vi "main_load_environment_check.vi"(10 "New working Dir":path) -> (1 "Structure":string, 2 "Valid?":bool, 3 "Endtime":string)   [LabVIEW 2019]
uses:
  <vilib>/regexp/Match Regular Expression.xnode
panel:
  out "Starttime":string
  out "Finished?":string
  out "Timesteps":i32[](array[numeric])
  # "*******************************************************************\nBiogas Plant Control\n\nAuthor: Paul Zügel\nGCSC-Frankfurt am Main 2020\n\n*******************************************************************"
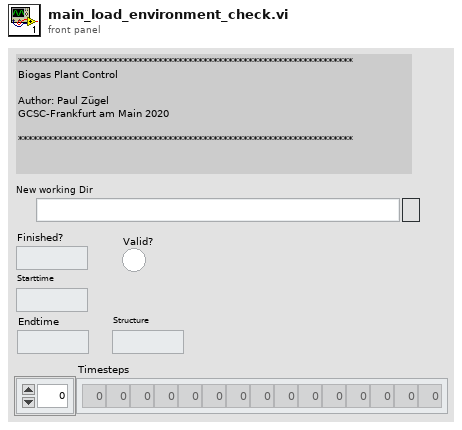
[diagram p1: front panel]
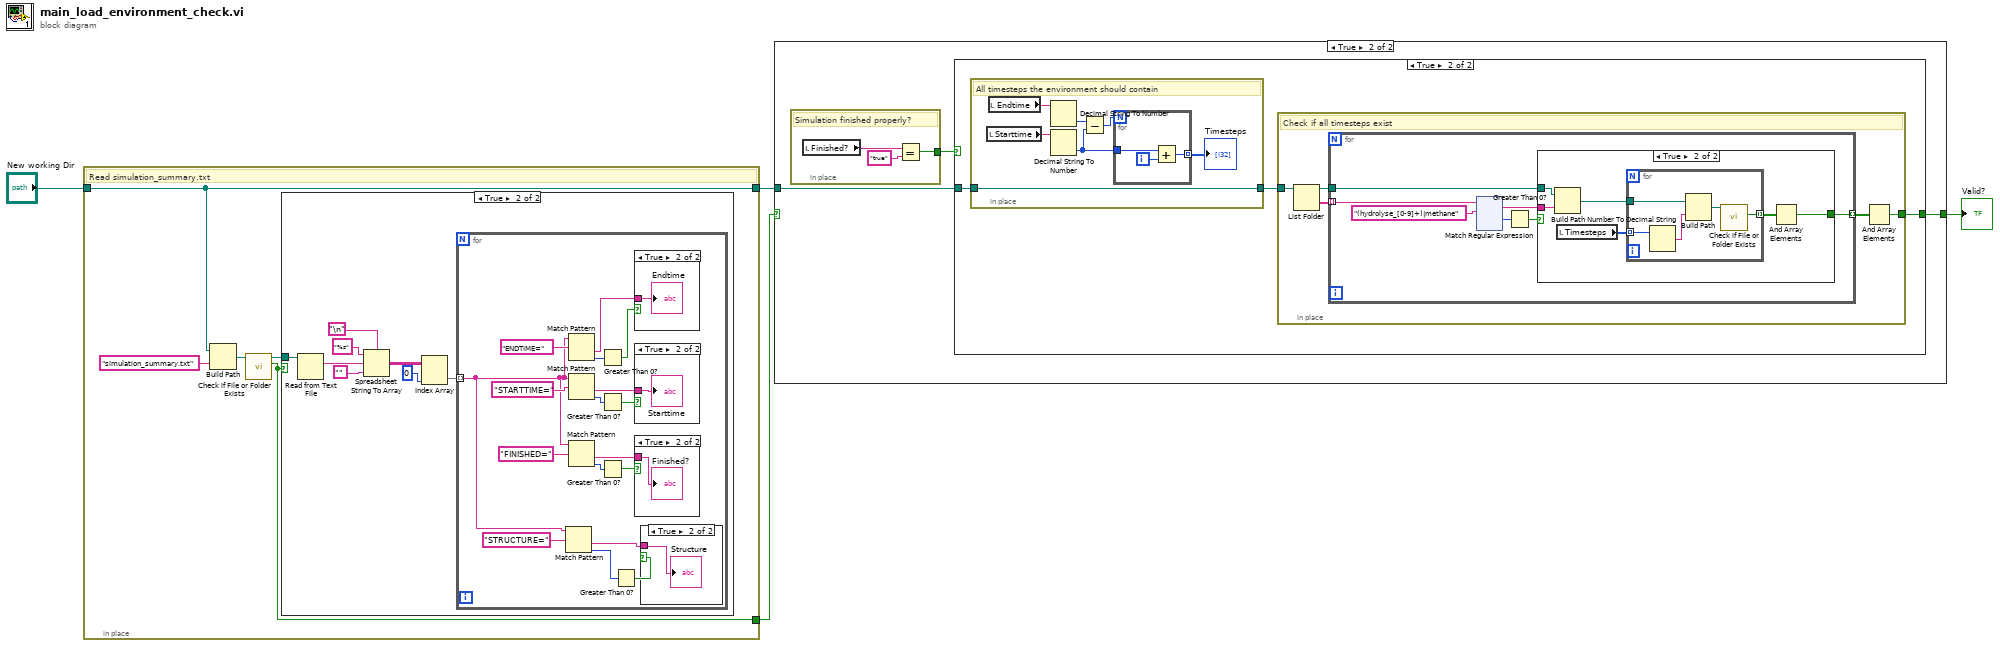
[diagram p0: block diagram]
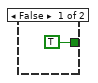
[diagram p4: hidden frame]
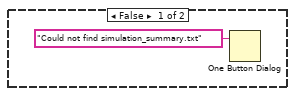
[diagram p5: hidden frame]
diagram:
  n1 = in-place {
    in-place-border: [w7] -> w1
    in-place-border: "New working Dir" -> [w5]
    in-place-border: [w5] -> w2
    # "Read simulation_summary.txt"
    n2 = Build Path(base path=w5, name or relative path="simulation_summary.txt") -> (appended path=w6:path)
    n3 = call <vilib>:"Check if File or Folder Exists.vi"("path"=w6) -> ("file or folder exists?"=w7:bool, "dup path"=w8:path)  [unwired: 8 in, 1 out]
    n4 = case shown="True" w7 {
      tunnel: w8 -> [_ w18]
      frame False {
        n5 = One Button Dialog(message="Could not find simulation_summary.txt") -> ()  [unwired: 1 in, 1 out]
      }
      frame True {
        n6 = Read from Text File(file (use dialog)=w18) -> (text=w17:string)  [unwired: 3 in, 3 out]
        n7 = Spreadsheet String To Array(delimiter (Tab)="\n", format string="%s", spreadsheet string=w17, array type (2D Dbl)="") -> (array=w11:string[][])
        n8 = Index Array(array=w11, index (col)=0 ("disabled index (col)")) -> (element=w12:string[])  [unwired: 1 in]
        n9 = for {
          tunnel: w12 -> [w19] mode=indexing
          n10 = Match Pattern(string=w19, regular expression="STRUCTURE=") -> (after substring=w22:string, offset past match=w21:i32)  [unwired: 1 in, 2 out]
          n11 = Match Pattern(string=w19, regular expression="ENDTIME=") -> (after substring=w30:string, offset past match=w25:i32)  [unwired: 1 in, 2 out]
          n12 = Match Pattern(string=w19, regular expression="STARTTIME=") -> (after substring=w32:string, offset past match=w27:i32)  [unwired: 1 in, 2 out]
          n13 = Match Pattern(string=w19, regular expression="FINISHED=") -> (after substring=w34:string, offset past match=w29:i32)  [unwired: 1 in, 2 out]
          n14 = Greater Than 0?(x=w25) -> (x > 0?=w24:bool)
          n15 = Greater Than 0?(x=w27) -> (x > 0?=w26:bool)
          n16 = Greater Than 0?(x=w29) -> (x > 0?=w28:bool)
          n17 = Greater Than 0?(x=w21) -> (x > 0?=w20:bool)
          n18 = case shown="True" w24 {
            tunnel: w30 -> [_ w39]
            frame False {
            }
            frame True {
              "Endtime" <- w39
            }
          }
          n19 = case shown="True" w26 {
            tunnel: w32 -> [_ w38]
            frame False {
            }
            frame True {
              "Starttime" <- w38
            }
          }
          n20 = case shown="True" w28 {
            tunnel: w34 -> [_ w37]
            frame False {
            }
            frame True {
              "Finished?" <- w37
            }
          }
          n21 = case shown="True" w20 {
            tunnel: w22 -> [_ w36]
            frame False {
            }
            frame True {
              "Structure" <- w36
            }
          }
        }
      }
    }
  }
  n22 = case shown="True" w1 {
    selector: w1 -> [w40 _]
    tunnel: [w40 w43] -> w4
    tunnel: w2 -> [_ w42]
    frame False {
    }
    frame True {
      n23 = in-place {
        in-place-border: [w196] -> w41
        # "Simulation finished properly?"
        n24 = local read "Finished?"() -> (w198:string)
        n25 = Equal?(x=w198, y="true") -> (x = y?=w196:bool)
      }
      n26 = case shown="True" w41 {
        selector: w41 -> [w44 _]
        tunnel: [w44 w47] -> w43
        tunnel: w42 -> [_ w45]
        frame False {
        }
        frame True {
          n27 = in-place {
            in-place-border: w45 -> [w50]
            in-place-border: [w50] -> w46
            # "All timesteps the environment should contain"
            n28 = local read "Starttime"() -> (w48:string)
            n29 = local read "Endtime"() -> (w49:string)
            n30 = Decimal String To Number(string=w49) -> (number=w54:i32)  [unwired: 2 in, 1 out]
            n31 = Decimal String To Number(string=w48) -> (number=w52:i32)  [unwired: 2 in, 1 out]
            n32 = Subtract(x=w54, y=w52) -> (x-y=w53:i32)
            n33 = for {
              N: w53 -> [_]
              tunnel: w52 -> [w56]
              tunnel: [w55] -> w51 mode=indexing
              i -> [w57]
              n34 = Add(x=w56, y=w57) -> (x+y=w55:i32)
            }
            "Timesteps" <- w51
          }
          n35 = in-place {
            in-place-border: [w62] -> w47
            in-place-border: w46 -> [w61]
            # "Check if all timesteps exist"
            n36 = List Folder(path=w61) -> (path out=w59:path, folder names=w60:string[])  [unwired: 3 in, 2 out]
            n37 = for {
              tunnel: w60 -> [w68] mode=indexing
              tunnel: w59 -> [w65]
              tunnel: [w63] -> w58 mode=indexing
              n38 = xnode "Match Regular Expression"("input string"=w68, "regular expression"="(hydrolyse_[0-9]+)|methane") -> ("whole match"=w64:string, "offset past match"=w67:i32)  [unwired: 4 in, 3 out]
              n39 = Greater Than 0?(x=w67) -> (x > 0?=w66:bool)
              n40 = case shown="True" w66 {
                tunnel: w65 -> [_ w76]
                tunnel: w64 -> [_ w75]
                tunnel: [TRUE w71] -> w63
                frame False {
                }
                frame True {
                  n41 = Build Path(base path=w76, name or relative path=w75) -> (appended path=w73:path)
                  n42 = local read "Timesteps"() -> (w74:i32[])
                  n43 = for {
                    tunnel: w74 -> [w80] mode=indexing
                    tunnel: w73 -> [w81]
                    tunnel: [w77] -> w72 mode=indexing
                    n44 = Number To Decimal String(number=w80) -> (decimal integer string=w79:string)  [unwired: 1 in]
                    n45 = Build Path(base path=w81, name or relative path=w79) -> (appended path=w78:path)
                    n46 = call <vilib>:"Check if File or Folder Exists.vi"("path"=w78) -> ("file or folder exists?"=w77:bool)  [unwired: 8 in, 2 out]
                  }
                  n47 = And Array Elements(Boolean array=w72) -> (logical AND=w71:bool)
                }
              }
            }
            n48 = And Array Elements(Boolean array=w58) -> (logical AND=w62:bool)
          }
        }
      }
    }
  }
  "Valid?" <- w4
